vi "Sweep Back and Forth.vi"(6 "Back and forth ?":bool, 7 "Index":i32, 8 "Step":dbl, 9 "Final":dbl, 10 "Initial":dbl) -> (2 "Last element ?":bool, 3 "element":dbl)   [LabVIEW 2016]
panel:
  out "Waveform Graph":dbl[](graph)
  out "Output array":dbl[](array[numeric])
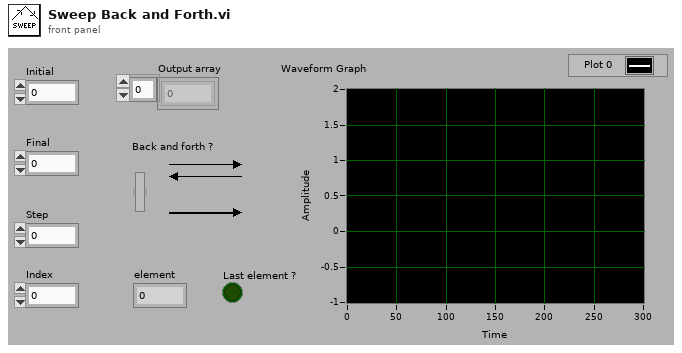
[diagram p1: front panel]
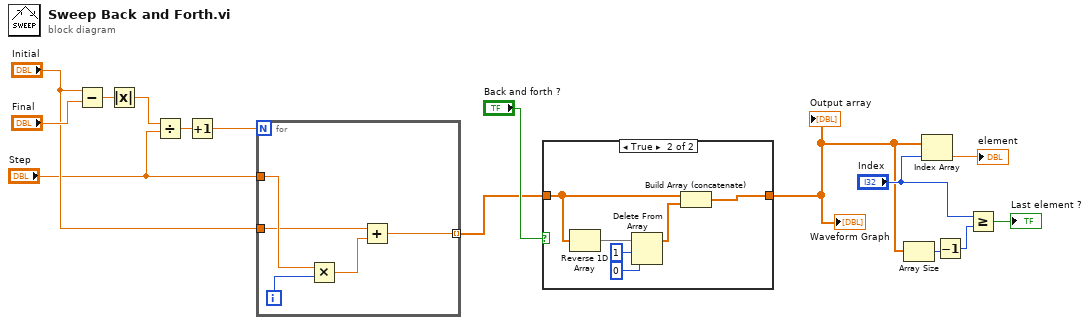
[diagram p0: block diagram]
diagram:
  n1 = Subtract(x="Initial", y="Final") -> (x-y=w14:dbl)
  n2 = Absolute Value(x=w14) -> (abs(x)=w13:dbl)
  n3 = Divide(x=w13, y="Step") -> (x/y=w12:dbl)
  n4 = Increment(x=w12) -> (x+1=w11:dbl)
  n5 = for {
    N: w11 -> [_]
    tunnel: "Initial" -> [w18]
    tunnel: "Step" -> [w20]
    tunnel: [w16] -> w7 mode=indexing
    i -> [w19]
    n6 = Multiply(x=w20, y=w19) -> (x*y=w17:dbl)
    n7 = Add(x=w18, y=w17) -> (x+y=w16:dbl)
  }
  n8 = case shown="True" "Back and forth ?" {
    tunnel: w7 -> [w21 w23]
    tunnel: [w21 w22] -> w1
    frame False {
    }
    frame True {
      n9 = Reverse 1D Array(array=w23) -> (reversed array=w24:dbl[])
      n10 = Delete From Array(array=w24, length=1, index=0) -> (array with subset deleted=w27:dbl[])  [unwired: 1 out]
      n11 = Build Array (concatenate)(w23, w27) -> (w22:dbl[])
    }
  }
  "Output array" <- w1
  "Waveform Graph" <- w1
  n12 = Array Size(array=w1) -> (size(s)=w4:i32)
  n13 = Index Array(array=w1, index="Index") -> (element=→"element":dbl)
  n14 = Decrement(x=w4) -> (x-1=w3:i32)
  n15 = Greater Or Equal?(x="Index", y=w3) -> (x >= y?=→"Last element ?":bool)
